vi "SpotGen Charge.vi"(5 "Charge Max SOC":sgl=90.0, 7 "Init":bool, 8 "Error In":errorcluster, 9 "FPGA Data":T1 {"SSG Active Current" format="%2.1f"; "PV Reactive Power (L1)" format="%2.1f"; "PV Reactive Power (L2)" format="%2.1f"; "PV Total Reactive Power" format="%2.1f"; "Gen Reactive Power (L1)" format="%2.1f"; "Gen Reactive Power (L2)" format="%2.1f"; "Gen Total Reactive Power" format="%2.1f"; "SSG Reactive Power (L1)" format="%2.1f"; "SSG Reactive Power (L2)" format="%2.1f"; "SSG Total Reactive Power" format="%2.1f"; "PV Total Current" format="%2.1f"; "PV Total Voltage" format="%2.1f"; "PV Active Power (L1)" format="%2.1f"; "PV Active Power (L2)" format="%2.1f"; "PV App Power (L1)" format="%2.1f"; "PV App Power (L2)" format="%2.1f"; "PV Total Active Power" format="%2.1f"; "PV Total App Power" format="%2.1f"; "PV Arms (L1)" format="%2.1f"; "PV Arms (L2)" format="%2.1f"; "PV Vrms (L1)" format="%2.1f"; "PV Vrms (L2)" format="%2.1f"; "Gen Total Current" format="%2.1f"; "SSG Total Current" format="%2.1f"; "Gen Total Voltage" format="%2.1f"; "SSG Total Voltage" format="%2.1f"; "Gen Active Power (L1)" format="%2.1f"; "Gen Active Power (L2)" format="%2.1f"; "SSG Active Power (L1)" format="%2.1f"; "SSG Active Power (L2)" format="%2.1f"; "Gen App Power (L1)" format="%2.1f"; "Gen App Power (L2)" format="%2.1f"; "SSG App Power (L1)" format="%2.1f"; "SSG App Power (L2)" format="%2.1f"; "Gen Total Active Power" format="%2.1f"; "Gen Total App Power" format="%2.1f"; "Gen Arms (L1)" format="%2.1f"; "Gen Arms (L2)" format="%2.1f"; "Gen Vrms (L1)" format="%2.1f"; "Gen Vrms (L2)" format="%2.1f"; "SSG Total Active Power" format="%2.1f"; "SSG Total App Power" format="%2.1f"; "SSG Arms (L1)" format="%2.1f"; "SSG Arms (L2)" format="%2.1f"; "SSG Vrms (L1)" format="%2.1f"; "SSG Vrms (L2)" format="%2.1f"}, 10 "ES System Data":T2={"Voltage"=0.0, "Current"=0.0, "SOC Avg"=0.0, "Faults"=0, "Alarms"=0, "# Strings"=0, "Max Temp"=0, "Min Temp"=0, "Max Cell Voltage"=0.0, "Min Cell Voltage"=0.0, "Energy Capacity"=0.0, "Energy Remaining"=0.0, "SOC Min"=0.0, "SOC Max"=0.0, "ES Fault"=FALSE, "String Select"=enum."3 Strings", "ES Com Fault"=FALSE, "SOH Avg"=0.0}) -> (0 "Error Out":errorcluster, 1 "PV Control":bool, 2 "Exit Charge Mode":bool, 3 "Current Setpoint":dbl)   [LabVIEW 2014]
uses:
  Controls/ES System Data.ctl
  Controls/StringSelector.ctl
  Controls/FPGA Data.ctl
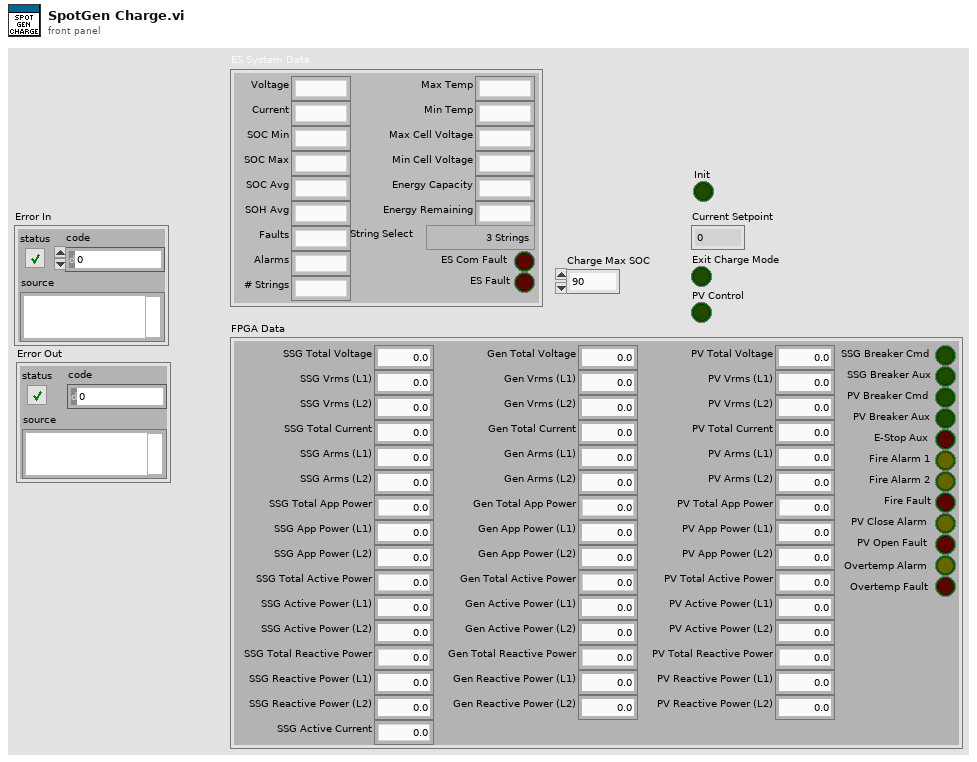
[diagram p1: front panel]
types:
  T1 = typedef "FPGA Data.ctl" = cluster{"Gen Total Voltage":dbl, "Gen Vrms (L1)":dbl, "Gen Vrms (L2)":dbl, "Gen Total Current":dbl, "Gen Arms (L1)":dbl, "Gen Arms (L2)":dbl, "Gen Total App Power":dbl, "Gen App Power (L1)":dbl, "Gen App Power (L2)":dbl, "Gen Total Active Power":dbl, "Gen Active Power (L1)":dbl, "Gen Active Power (L2)":dbl, "Gen Total Reactive Power":dbl, "Gen Reactive Power (L1)":dbl, "Gen Reactive Power (L2)":dbl, "SSG Total Voltage":dbl, "SSG Vrms (L1)":dbl, "SSG Vrms (L2)":dbl, "SSG Total Current":dbl, "SSG Arms (L1)":dbl, "SSG Arms (L2)":dbl, "SSG Total App Power":dbl, "SSG App Power (L1)":dbl, "SSG App Power (L2)":dbl, "SSG Total Active Power":dbl, "SSG Active Power (L1)":dbl, "SSG Active Power (L2)":dbl, "SSG Total Reactive Power":dbl, "SSG Reactive Power (L1)":dbl, "SSG Reactive Power (L2)":dbl, "PV Total Voltage":dbl, "PV Vrms (L1)":dbl, "PV Vrms (L2)":dbl, "PV Total Current":dbl, "PV Arms (L1)":dbl, "PV Arms (L2)":dbl, "PV Total App Power":dbl, "PV App Power (L1)":dbl, "PV App Power (L2)":dbl, "PV Total Active Power":dbl, "PV Active Power (L1)":dbl, "PV Active Power (L2)":dbl, "PV Total Reactive Power":dbl, "PV Reactive Power (L1)":dbl, "PV Reactive Power (L2)":dbl, "SSG Breaker Cmd":bool, "SSG Breaker Aux":bool, "PV Breaker Cmd":bool, "PV Breaker Aux":bool, "E-Stop Aux":bool, "Fire Alarm 1":bool, "Fire Alarm 2":bool, "Fire Fault":bool, "PV Close Alarm":bool, "SSG Active Current":dbl, "Overtemp Alarm":bool, "Overtemp Fault":bool, "PV Open Fault":bool}
  T2 = typedef "ES System Data.ctl" = cluster{"Voltage":sgl, "Current":sgl, "SOC Avg":sgl, "Faults":u16, "Alarms":u16, "# Strings":u16, "Max Temp":i16, "Min Temp":i16, "Max Cell Voltage":sgl, "Min Cell Voltage":sgl, "Energy Capacity":sgl, "Energy Remaining":sgl, "SOC Min":sgl, "SOC Max":sgl, "ES Fault":bool, "String Select":T3, "ES Com Fault":bool, "SOH Avg":sgl}
  T3 = typedef "StringSelector.ctl" = enum16{"1 String (1)", "1 String (2)", "1 String (3)", "2 Strings (1 2)", "2 Strings (2 3)", "2 Strings (1 3)", "3 Strings"}
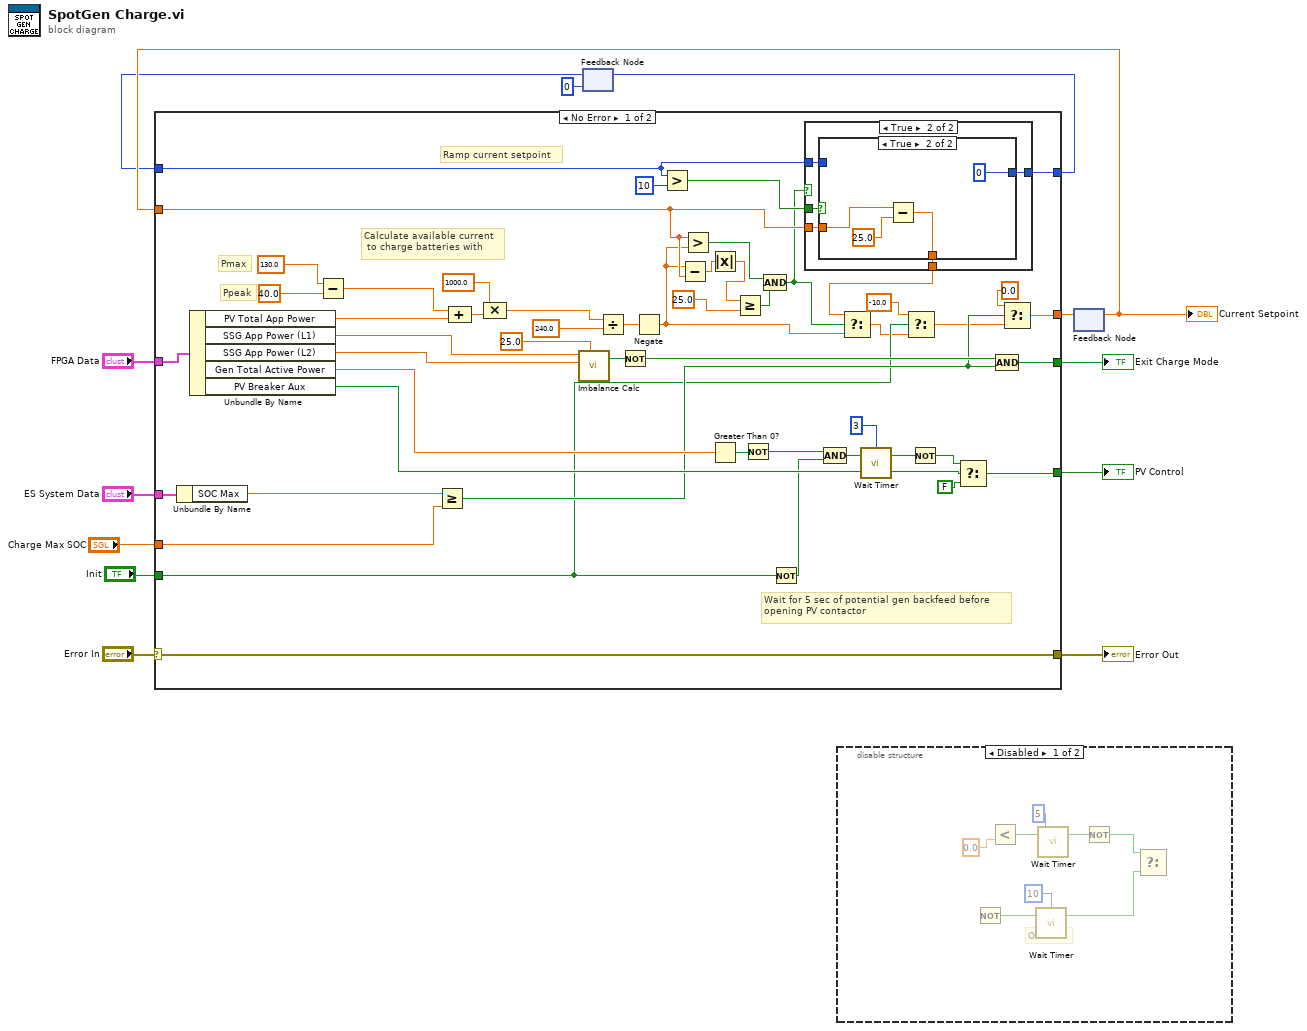
[diagram p0: block diagram]
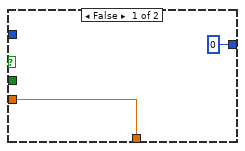
[diagram p3: hidden frame]
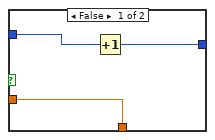
[diagram p4: hidden frame]
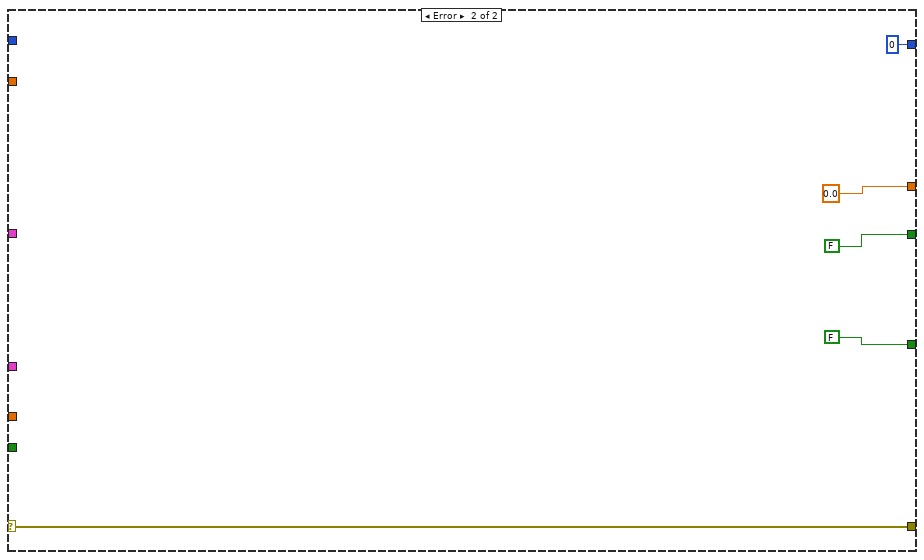
[diagram p5: hidden frame]
diagram:
  n1 = feedback #1(u16 0) -> (w3:i32)
  n2 = disable-structure shown="Disabled" {
    frame Disabled {
      # "On filter"
      n3 = Not() -> (x=w20:bool, .not. x?=w19:bool)
      n4 = Less?(y=0.0) -> (x < y?=w16:bool)  [unwired: 1 in]
      n5 = call "Wait Timer.vi"("Boolean In"=w19, "Timer"=u32 10) -> ("Boolean Out"=w22:bool)  [unwired: 3 in]
      n6 = call "Wait Timer.vi"("Boolean In"=w16, "Timer"=u32 5) -> ("Boolean Out"=w15:bool)  [unwired: 3 in]
      n7 = Not(x=w15) -> (.not. x?=w23:bool)
      n8 = Select(t=w23, f=w22) -> (s=w21:bool)  [unwired: 1 out]
    }
    frame Enabled {
    }
  }
  n9 = feedback #2() -> (w4:dbl)  [unwired: 1 in]
  "Current Setpoint" <- w4
  n10 = case shown="No Error" "Error In" {
    selector: "Error In" -> [w64 w93]
    tunnel: "FPGA Data" -> [w65 _]
    tunnel: [w46 0.0] -> w5
    tunnel: [w64 w93] -> w11
    tunnel: "ES System Data" -> [w60 _]
    tunnel: [w53 FALSE] -> w9
    tunnel: [w61 FALSE] -> w8
    tunnel: "Init" -> [w29 _]
    tunnel: "Charge Max SOC" -> [w44 _]
    tunnel: w4 -> [w37 _]
    tunnel: w3 -> [w32 _]
    tunnel: [w38 0] -> w1
    frame No Error {
      # "Ramp current setpoint"
      # "Calculate available current\n to charge batteries with"
      # "Wait for 5 sec of potential gen backfeed before\nopening PV contactor"
      # "Ppeak"
      # "Pmax"
      n11 = Unbundle By Name(w60) -> ("SOC Max"=w43:sgl)
      n12 = Unbundle By Name(w65) -> ("PV Total App Power"=w71:dbl, "SSG App Power (L1)"=w70:dbl, "SSG App Power (L2)"=w69:dbl, "Gen Total Active Power"=w56:dbl, "PV Breaker Aux"=w55:bool)
      n13 = Subtract(x=130.0, y=40.0) -> (x-y=w72:dbl)
      n14 = Greater Or Equal?(x=w43, y=w44) -> (x >= y?=w42:bool)
      n15 = Compound Arithmetic op=ADD(w72, w71) -> (w59:dbl)
      n16 = Compound Arithmetic op=MULTIPLY(1000.0 ("value"), w59) -> (w58:dbl)
      n17 = call "Imbalance Calc.vi"("A"=w70, "B"=w69, "X"=25.0) -> ("|A-B|>X?"=w67:bool)  [unwired: 3 in]
      n18 = Divide(x=w58, y=240.0 ("upper limit")) -> (x/y=w62:dbl)
      n19 = Not(x=w67) -> (.not. x?=w66:bool)
      n20 = Negate(x=w62) -> (-x=w33:dbl)
      n21 = Greater?(x=w32, y=u16 10) -> (0:w40:bool)
      n22 = Subtract(x=w33, y=w37) -> (x-y=w25:dbl)
      n23 = Greater?(x=w37, y=w33) -> (0:w34:bool)
      n24 = Absolute Value(x=w25) -> (abs(x)=w24:dbl)
      n25 = Greater Than 0?(x=w56) -> (x > 0?=w52:bool)
      n26 = Greater Or Equal?(x=w24, y=25.0) -> (x >= y?=w35:bool)
      n27 = Not(x=w52) -> (.not. x?=w48:bool)
      n28 = Compound Arithmetic op=AND(w34, w35) -> (w31:bool)
      n29 = Not(x=w29) -> (.not. x?=w30:bool)
      n30 = case shown="True" w31 {
        tunnel: w40 -> [_ w81]
        tunnel: [w75 w80] -> w39
        tunnel: [0 w79] -> w38
        tunnel: w37 -> [w75 w78]
        tunnel: w32 -> [_ w77]
        frame False {
        }
        frame True {
          n31 = case shown="True" w81 {
            tunnel: [w82 0] -> w79
            tunnel: w77 -> [w83 _]
            tunnel: w78 -> [w84 w86]
            tunnel: [w84 w87] -> w80
            frame False {
              n32 = Increment(x=w83) -> (x+1=w82:i32)
            }
            frame True {
              n33 = Subtract(x=w86, y=25.0 ("x")) -> (x-y=w87:dbl)
            }
          }
        }
      }
      n34 = Compound Arithmetic op=AND(w48, w30) -> (w47:bool)
      n35 = Select(t=w39, s=w31, f=w33) -> (s? t:f=w27:dbl)
      n36 = call "Wait Timer.vi"("Boolean In"=w47, "Timer"=u32 3) -> ("Boolean Out"=w50:bool)  [unwired: 3 in]
      n37 = Select(t=-10.0 ("f"), s=w29, f=w27) -> (s? t:f=w26:dbl)
      n38 = Not(x=w50) -> (.not. x?=w49:bool)
      n39 = Select(t=w49, s=w55, f=FALSE) -> (s? t:f=w53:bool)
      n40 = Compound Arithmetic op=AND(w66, w42) -> (w61:bool)
      n41 = Select(t=0.0, s=w42, f=w26) -> (s? t:f=w46:dbl)
    }
    frame Error {
    }
  }
  "Error Out" <- w11
  "Exit Charge Mode" <- w8
  "PV Control" <- w9
  n42 = feedback-in #1(w1) -> ()
  n43 = feedback-in #2(w5) -> ()
